vi "Configure DC Power Session.vi"(8 "error in":errorcluster, 9 "measurement configuration":T1={"pin_names"=[], "voltage_level"=6.0, "voltage_level_range"=6.0, "current_limit"=0.01, "current_limit_range"=0.01, "source_delay"=0.0}, 10 "channel list":string caption="channel name", 11 "instrument handle":refnum<k15>) -> (0 "error out":errorcluster, 3 "instrument handle":refnum<k15>)   [LabVIEW 2020, in "NIDCPowerSourceDCVoltage.lvlib"]
doc: "Configures the DC power sessions to be used in the measurement logic."
uses:
  Measurement Configuration.ctl
  <instrlib>/niDCPower/nidcpower.llb/niDCPower Source Mode.ctl
  <instrlib>/niDCPower/nidcpower.llb/niDCPower Output Function.ctl
  NIDCPowerSourceDCVoltage.lvlib
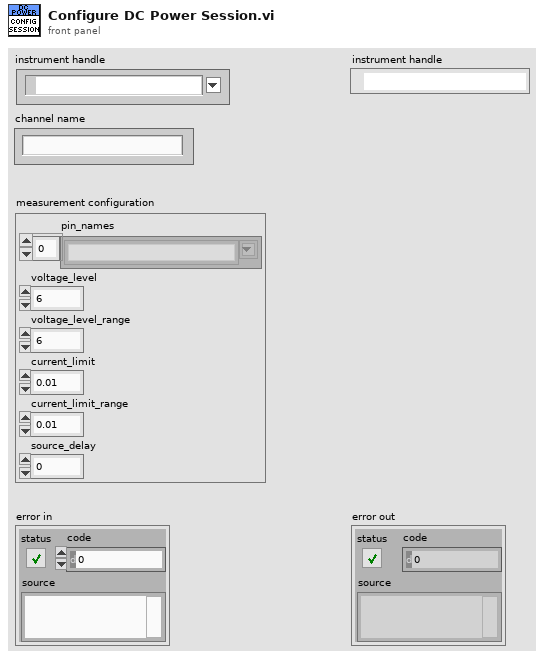
[diagram p1: front panel]
types:
  T1 = typedef "NIDCPowerSourceDCVoltage.lvlib/Measurement Configuration.ctl" = cluster{"pin_names":string[], "voltage_level":dbl, "voltage_level_range":dbl, "current_limit":dbl, "current_limit_range":dbl, "source_delay":dbl}
  T2 = typedef "niDCPower Output Function.ctl" = i32
  T3 = typedef "niDCPower Source Mode.ctl" = i32
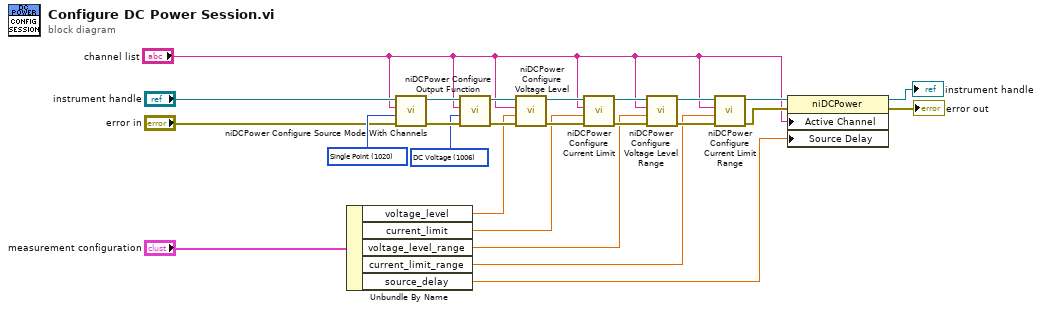
[diagram p0: block diagram]
diagram:
  w12 = T2 1006 items=["DC Voltage"=1006, "DC Current"=1007, "Pulse Voltage"=1049, "Pulse Current"=1050] ("output function")
  w13 = T3 1020 items=["Single Point"=1020, "Sequence"=1021] ("source mode")
  n1 = Unbundle By Name("measurement configuration") -> ("voltage_level"=w11:dbl, "current_limit"=w10:dbl, "voltage_level_range"=w8:dbl, "current_limit_range"=w7:dbl, "source_delay"=w6:dbl)
  n2 = call <instrlib>:"niDCPower Configure Source Mode With Channels.vi"("error in (no error)"="error in", "source mode"=w13, "channel name"="channel list", "instrument handle"="instrument handle") -> ("error out"=w23:errorcluster, "instrument handle out"=w22:refnum<k15>)  [unwired: 6 in]
  n3 = call <instrlib>:"niDCPower Configure Output Function.vi"("error in (no error)"=w23, "output function"=w12, "channel name"="channel list", "instrument handle"=w22) -> ("error out"=w14:errorcluster, "instrument handle out"=w15:refnum<k15>)  [unwired: 6 out]
  n4 = call <instrlib>:"niDCPower Configure Voltage Level.vi"("error in (no error)"=w14, "voltage level"=w11, "channel name"="channel list", "instrument handle"=w15) -> ("error out"=w24:errorcluster, "instrument handle out"=w25:refnum<k15>)  [unwired: 6 out]
  n5 = call <instrlib>:"niDCPower Configure Current Limit.vi"("error in (no error)"=w24, "current limit"=w10, "channel name"="channel list", "instrument handle"=w25) -> ("error out"=w21:errorcluster, "instrument handle out"=w20:refnum<k15>)  [unwired: 1 in, 5 out]
  n6 = call <instrlib>:"niDCPower Configure Voltage Level Range.vi"("error in (no error)"=w21, "voltage level range"=w8, "channel name"="channel list", "instrument handle"=w20) -> ("error out"=w19:errorcluster, "instrument handle out"=w18:refnum<k15>)  [unwired: 6 out]
  n7 = call <instrlib>:"niDCPower Configure Current Limit Range.vi"("error in (no error)"=w19, "current limit range"=w7, "channel name"="channel list", "instrument handle"=w18) -> ("error out"=w16:errorcluster, "instrument handle out"=w17:refnum<k15>)  [unwired: 6 out]
  n8 = property class="niDCPower"(reference=w17, error in=w16, "Active Channel"="channel list", "Source Delay"=w6) -> (reference out=→"instrument handle":refnum<k15>, error out=→"error out":errorcluster)
